vi "addFileCategory.vi"(1 "VarableID":T1) -> ()   [LabVIEW 2010]
uses:
  VarableID.ctl
  VarableStruct.ctl
  GlobalCostants.vi
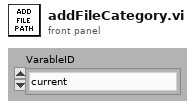
[diagram p1: front panel]
types:
  T1 = typedef "VarableID.ctl" = enum16{"current", "voltage", "power", "PF"}
  T2 = typedef "VarableStruct.ctl" = cluster{"Name":string, "StorageRefnum":refnum<file>, "Command":string, "IsDetecting":bool, "VarableID":T1}
  T3 = enum16{"open", "replace", "create", "open or create", "replace or create", "replace or create with confirmation"}
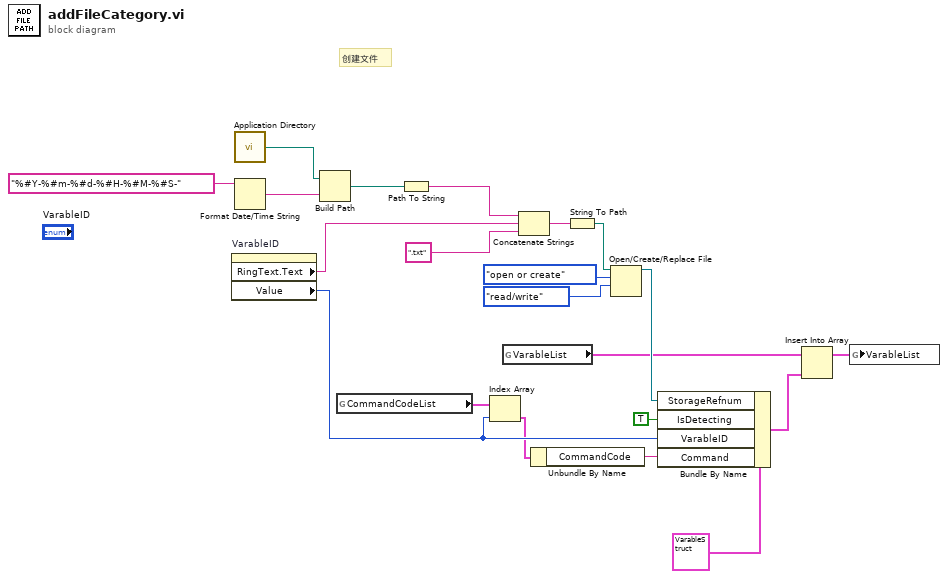
[diagram p0: block diagram]
diagram:
  # "创建文件"
  n1 = property on="VarableID" class="Enum (strict)"() -> ("RingText.Text"=w11:string, "Value"=w3:enum16{"current", "voltage", "power", "PF"})  [unwired: 2 in, 2 out]
  n2 = call <vilib>:"Application Directory.vi"() -> ("Application Directory"=w19:path)
  n3 = Format Date/Time String(time format string (%c)="%#Y-%#m-%#d-%#H-%#M-%#S-") -> (date/time string=w20:string)  [unwired: 2 in]
  n4 = Build Path(base path=w19, name or relative path=w20) -> (appended path=w21:path)
  n5 = global read "GlobalCostants.vi" "CommandCodeList"() -> (w4:cluster{"CommandCode":string, "VarableID":T1}[])
  n6 = Path To String(path=w21) -> (string=w13:string)
  n7 = Index Array(array=w4, index=w3) -> (element=w2:cluster{"CommandCode":string, "VarableID":T1})
  n8 = global read "GlobalCostants.vi" "VarableList"() -> (w7:T2[])
  n9 = Concatenate Strings(w13, w11, ".txt" ("字符串")) -> (w15:string)
  n10 = Unbundle By Name(w2) -> ("CommandCode"=w1:string)
  n11 = String To Path(string=w15) -> (path=w14:path)
  n12 = Open/Create/Replace File(file path (use dialog)=w14, operation (0:open)=T3."open or create" ("操作(0:open)"), access (0:read/write)=enum16{"read/write", "read-only", "write-only"}."read/write" ("权限(0:read/write)")) -> (refnum out=w10:refnum<file>)  [unwired: 3 in, 2 out]
  n13 = Bundle By Name(cluster=T2 {"Name"="", "StorageRefnum"=refnum, "Command"="", "IsDetecting"=FALSE, "VarableID"=enum."current"} ("element"), "StorageRefnum"=w10, "IsDetecting"=TRUE, "VarableID"=w3, "Command"=w1) -> (w5:T2)
  n14 = Insert Into Array(array=w7, new element=w5) -> (w6:T2[])  [unwired: 1 in]
  n15 = global write "GlobalCostants.vi" "VarableList"(w6) -> ()
